vi "fake_camera.vi"() -> ()   [LabVIEW 2013]
uses:
  Global.vi
panel:
  in  "stop":bool
  in  "Tab Control":enum32{"Camera", "Settings"}(tab)
  in  "Pause":bool
  out "Image":T1(plugin-control)
  in  "Zoom":bool
  out "image":i32=7
  in  "max":i32=35000
  in  "min":i32=-35000
  out "Saving":bool
  in  "Exposure (ms)":i32=1000
  in  "Colour":u32(ring) items=["Grayscale", "Binary", "Gradient", "Rainbow", "Temperature", "User Defined"]
  out "Image Pixels (I16)":i16[][](array[numeric])=[[-29428, 11281, -2474, 30123, 9459, 1352, 24347, 32163], [-22381, -12034, 23578, -12849, 4549, 1086, -258, 14251], [-1433, 354, 7138, 14989, 9369, 10323, 31605, -19146], [15785, -3832, 17788, 3481, 31762, 11344, 21057, 6271], [-29804, 21898, -22162, 315, 20832, 27656, -25287, 17601], [-24529, 30912, -2445, 27456, -13882, 29588, -9856, -4296], [16108, 15514, -14038, -19065, 26211, -6562, -3334, 32401], [-29375, -23870, -14001, -3391, 9091, -22040, 29881, -14750]]
  out "error out":errorcluster
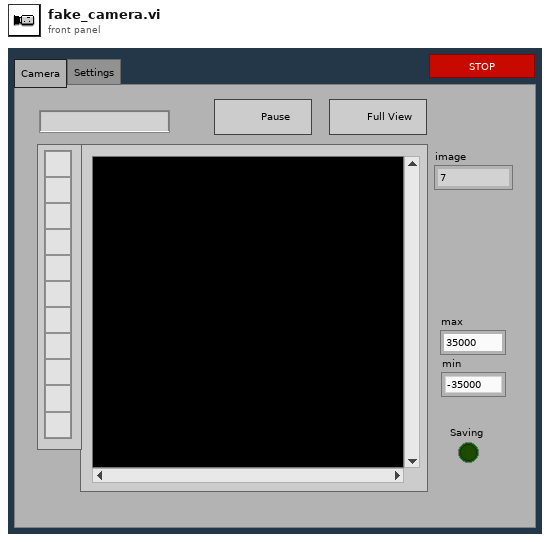
[diagram p1: front panel]
types:
  T1 = typedef "IMAQ Image.ctl" = refnum<image>
  T2 = typedef "Image Type" = u32
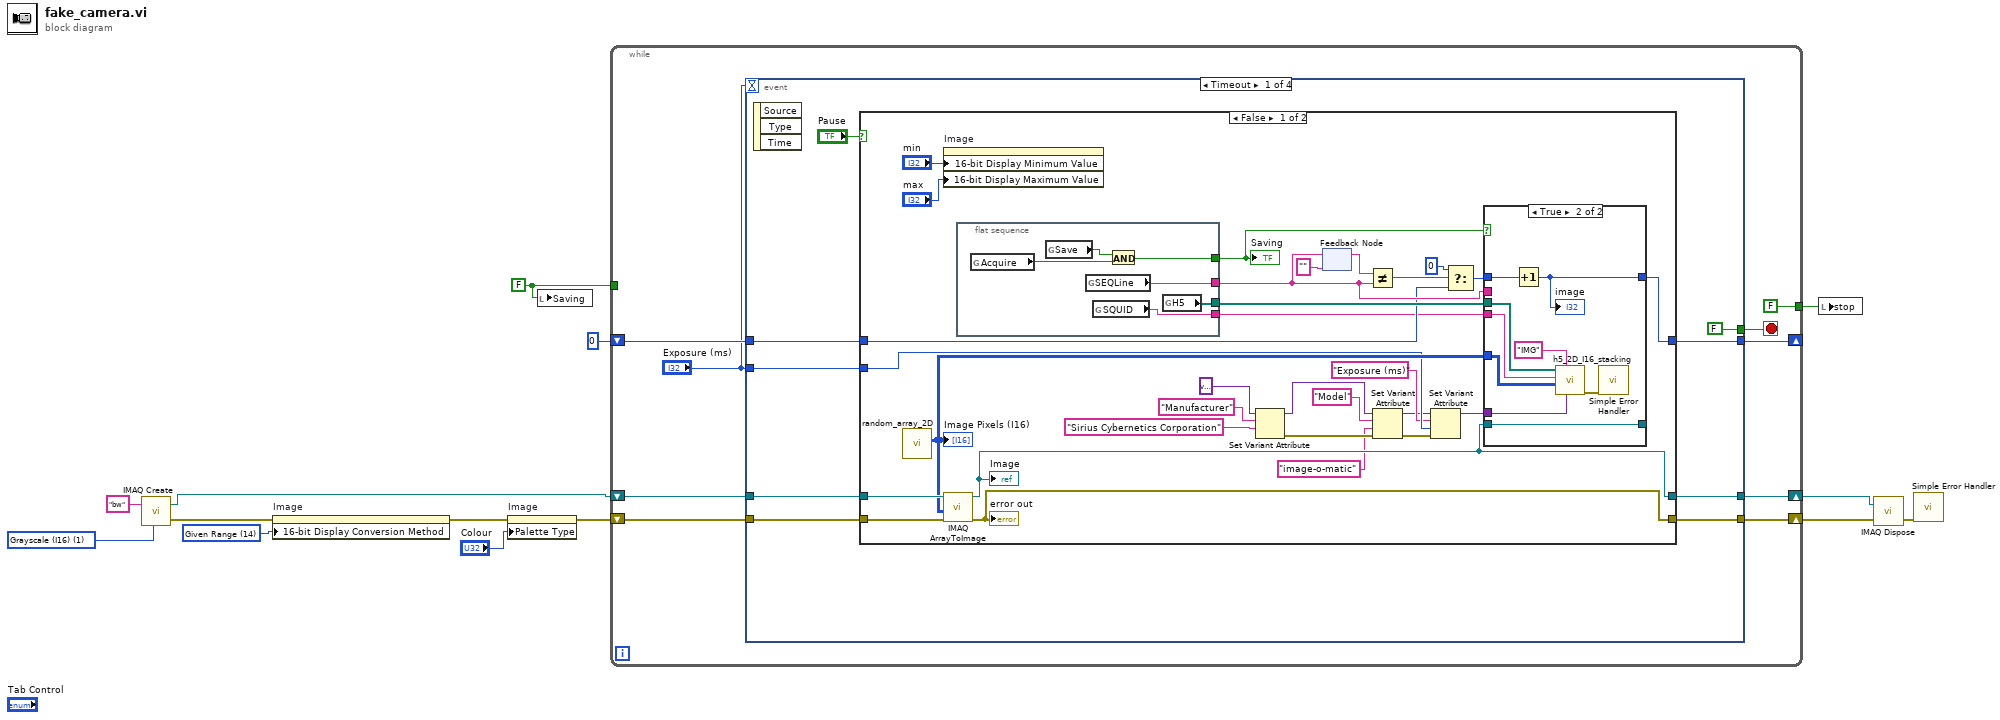
[diagram p0: block diagram]
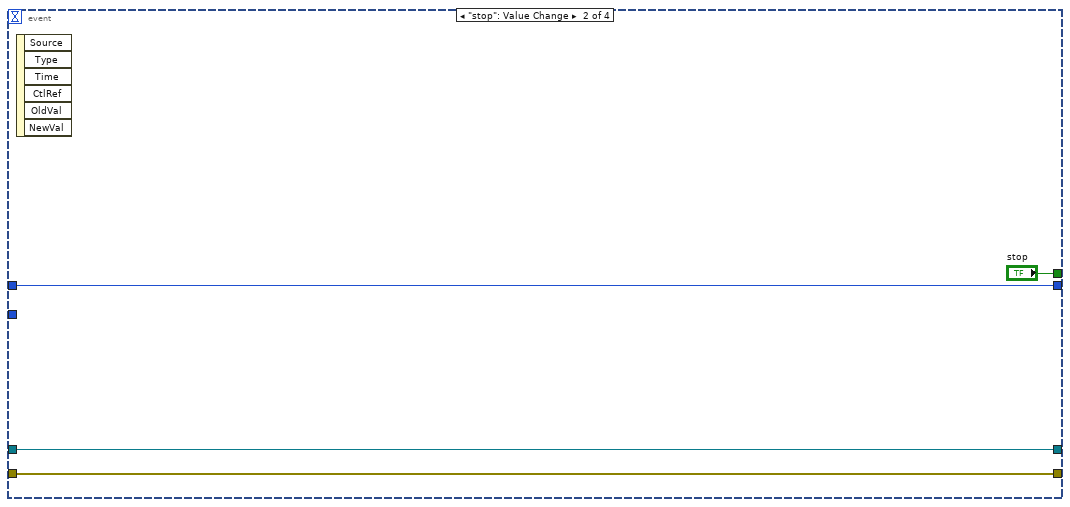
[diagram p4: hidden frame]
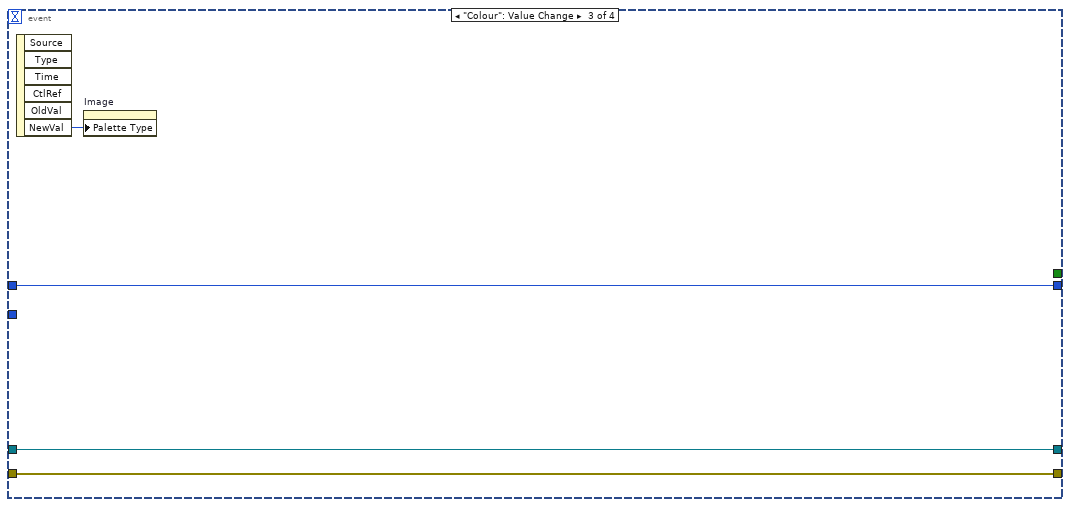
[diagram p5: hidden frame]
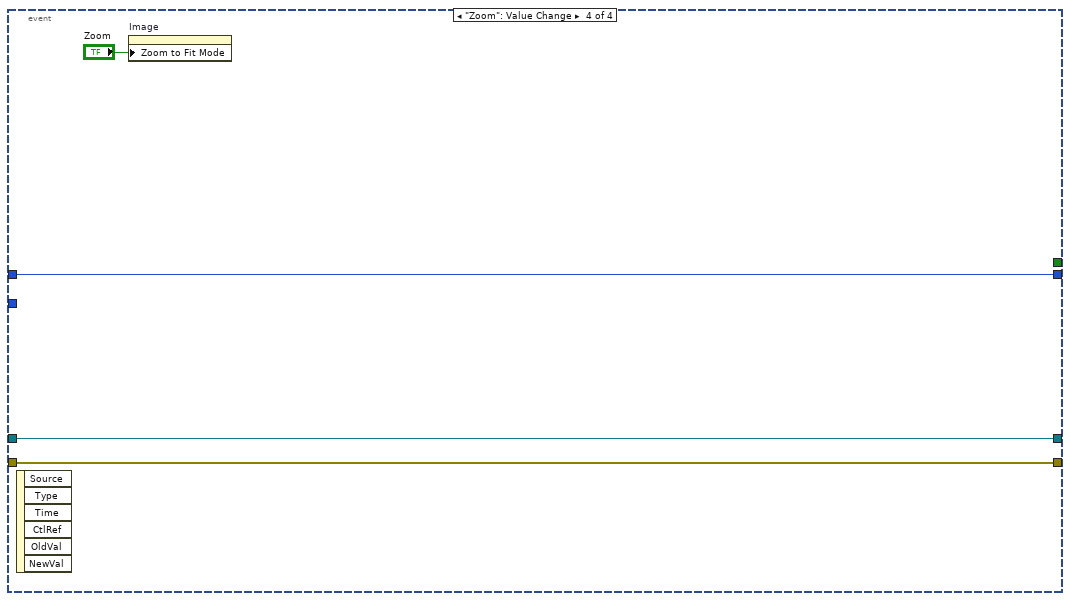
[diagram p6: hidden frame]
diagram:
  w1 = FALSE ("Saving")
  w12 = u32 14 items=["Default"=10, "Most Significant Bits"=11, "Full Dynamic"=12, "Downshift"=13, "Given Range"=14, "90% Dynamic"=15, "Given Percent Range"=16] ("16-bit Display Mapping:Conversion Method")
  w14 = T2 1 items=["Grayscale (U8)", "Grayscale (I16)", "Grayscale (SGL)", "Complex (CSG)", "RGB (U32)", "HSL (U32)", "RGB (U64)", "Grayscale (U16)"] ("Image Type")
  n1 = call "IMAQ Create"("Image Name"="bw", "Image Type"=w14) -> ("New Image"=w5:T1, "error out"=w4:errorcluster)  [unwired: 3 in]
  n2 = property on="Image" class="ImageControl"(error in=w4, "16-bit Display Conversion Method"=w12) -> (error out=w9:errorcluster)  [unwired: 1 in, 1 out]
  n3 = property on="Image" class="ImageControl"(error in=w9, "Palette Type"="Colour") -> (error out=w3:errorcluster)  [unwired: 1 in, 1 out]
  n4 = local write "Saving"(w1) -> ()
  n5 = while {
    shift-right: [w23] -> w6
    shift-left: w5 -> [w21]
    shift-right: [w20] -> w2
    shift-left: w3 -> [w19]
    shift-right: [w17] -> _
    shift-left: 0 ("Timeout (ms) 2") -> [w18]
    tunnel: [FALSE ("stop")] -> w7
    tunnel: w1 -> [_]
    stop <- w22 stop-if-true
    n6 = event shown="[0] Timeout" {
      selector: _ -> [_ _ _ _]
      dyn-events: _ -> [_ _ _ _]
      timeout: "Exposure (ms)" -> [_ _ _ _]
      tunnel: w21 -> [w32 w85 w88 w93]
      tunnel: [w30 w85 w88 w93] -> w23
      tunnel: [FALSE ("Stop") "stop" _ _] -> w22
      tunnel: [w29 w86 w89 w92] -> w20
      tunnel: w19 -> [w31 w86 w89 w92]
      tunnel: w18 -> [w28 w84 w87 w91]
      tunnel: [w27 w84 w87 w91] -> w17
      tunnel: "Exposure (ms)" -> [w24 _ _ _]
      event Timeout {
        n7 = event-data() -> ()  [unwired: 1 in, 3 out]
        n8 = case shown="False" "Pause" {
          tunnel: w32 -> [w50 w82]
          tunnel: w31 -> [w51 w81]
          tunnel: [w49 w82] -> w30
          tunnel: [w48 w81] -> w29
          tunnel: w28 -> [w55 w80]
          tunnel: [w62 w80] -> w27
          tunnel: w24 -> [w37 _]
          frame False {
            n9 = call "random_array_2D.vi"() -> ("array"=w45:i16[][])  [unwired: 11 in]
            "Image Pixels (I16)" <- w45
            n10 = property on="Image" class="ImageControl"("16-bit Display Minimum Value"="min", "16-bit Display Maximum Value"="max") -> ()  [unwired: 2 in, 2 out]
            n11 = call "IMAQ ArrayToImage"("error in (no error)"=w51, "Image Pixels (I16)"=w45, "Image"=w50) -> ("error out"=w48:errorcluster, "Image Out"=w49:T1)  [unwired: 7 in]
            "Image" <- w49
            "error out" <- w48
            n12 = flat-sequence {
              tunnel: [w68] -> w59
              tunnel: [w66] -> w57
              tunnel: [w67] -> w58
              tunnel: [w65] -> w52
              frame #0 {
                n13 = global read "Global.vi" "Acquire"() -> (w63:bool)
                n14 = global read "Global.vi" "Save"() -> (w64:bool)
                n15 = global read "Global.vi" "SEQLine"() -> (w66:string)
                n16 = global read "Global.vi" "SQUID"() -> (w65:string)
                n17 = And(x=w64, y=w63) -> (x .and. y?=w68:bool)
                n18 = global read "Global.vi" "H5"() -> (w67:path[])
              }
            }
            n19 = Set Variant Attribute(Variant=variant ("variant"), name="Manufacturer", value="Sirius Cybernetics Corporation" ("Make")) -> (Variant out=w42:variant, error out=w43:errorcluster)  [unwired: 1 in, 1 out]
            n20 = feedback #1("" ("Seq")) -> (w60:string)
            n21 = feedback-in #1(w57) -> ()
            n22 = Not Equal?(x=w60, y=w57) -> (x != y?=w53:bool)
            n23 = Set Variant Attribute(Variant=w42, name="Model", value="image-o-matic" ("name"), error in=w43) -> (Variant out=w34:variant, error out=w35:errorcluster)  [unwired: 1 out]
            n24 = Set Variant Attribute(Variant=w34, name="Exposure (ms)", value=w37, error in=w35) -> (Variant out=w33:variant)  [unwired: 2 out]
            n25 = Select(t=0 ("Timeout (ms) 2"), s=w53, f=w55) -> (s? t:f=w56:i32)
            n26 = case shown="True" w59 {
              tunnel: [w70 w77] -> _
              tunnel: w49 -> [w70 w77]
              tunnel: w56 -> [w69 w79]
              tunnel: [w69 w78] -> w62
              tunnel: w58 -> [_ w76]
              tunnel: w57 -> [_ _]
              tunnel: w52 -> [_ w74]
              tunnel: w45 -> [_ w72]
              tunnel: w33 -> [_ w71]
              frame False {
              }
              frame True {
                n27 = Increment(x=w79) -> (x+1=w78:i32)
                "image" <- w78
                n28 = call "h5_2D_I16_stacking.vi"("Attributes"=w71, "TYPE"="IMG", "2D I16"=w72, "SQUID"=w74, "H5"=w76) -> ("error out"=w73:errorcluster)  [unwired: 5 in, 1 out]
                n29 = call <vilib>:"Simple Error Handler.vi"("error in (no error)"=w73) -> ()  [unwired: 4 in, 5 out]
              }
            }
            "Saving" <- w59
          }
          frame True {
          }
        }
      }
      event "stop": Value Change {
        n30 = event-data() -> ()  [unwired: 1 in, 6 out]
      }
      event "Colour": Value Change {
        n31 = event-data() -> ("NewVal"=w90:u32)  [unwired: 1 in, 5 out]
        n32 = property on="Image" class="ImageControl"("Palette Type"=w90) -> ()  [unwired: 2 in, 2 out]
      }
      event "Zoom": Value Change {
        n33 = event-data() -> ()  [unwired: 1 in, 6 out]
        n34 = property on="Image" class="ImageControl"("Zoom to Fit Mode"="Zoom") -> ()  [unwired: 2 in, 2 out]
      }
    }
  }
  n35 = local write "stop"(w7) -> ()
  n36 = call "IMAQ Dispose"("Image"=w6, "error in (no error)"=w2) -> ("error out"=w11:errorcluster)  [unwired: 4 in]
  n37 = call <vilib>:"Simple Error Handler.vi"("error in (no error)"=w11) -> ()  [unwired: 4 in, 5 out]
